vi "GetCalibData.vi"(8 "error in (no error)":errorcluster, 11 "BME68x in":refnum<class "BME680.lvclass">) -> (0 "error out":errorcluster, 3 "BME68x out":refnum<class "BME680.lvclass">)   [LabVIEW 2022 SP3, in "BME680.lvlib" / "BME680.lvclass"]
uses:
  BME680.lvclass
  BME680.lvclass/BME680.ctl
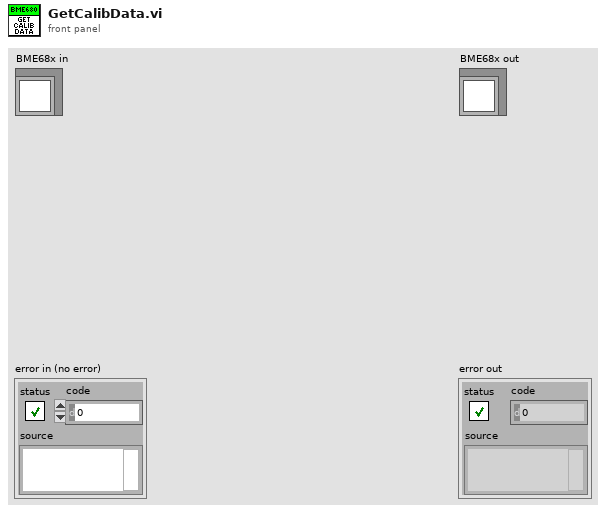
[diagram p1: front panel]
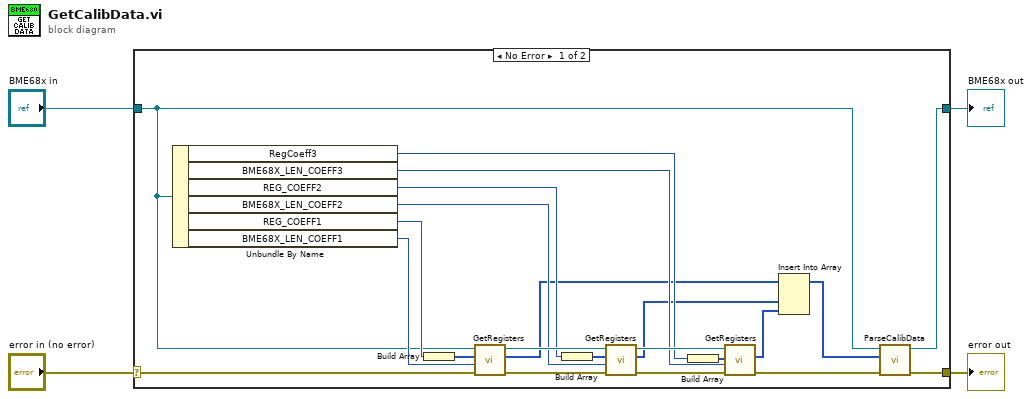
[diagram p0: block diagram]
diagram:
  n1 = case shown="No Error" "error in (no error)" {
    selector: "error in (no error)" -> [w26 w28]
    tunnel: [w11 w28] -> w3
    tunnel: [w5 w27] -> w1
    tunnel: "BME68x in" -> [w6 w27]
    frame No Error {
      n2 = Unbundle By Name(w6) -> ("RegCoeff3"=w15:u8, "BME68X_LEN_COEFF3"=w13:u8, "REG_COEFF2"=w18:u8, "BME68X_LEN_COEFF2"=w17:u8, "REG_COEFF1"=w24:u8, "BME68X_LEN_COEFF1"=w25:u8)
      n3 = Build Array(w24) -> (w23:u8[])
      n4 = call-dynamic "GetRegisters.vi"("error in (no error)"=w26, "Lenght"=w25, "Addr"=w23, "BME680 in"=w6) -> ("error out"=w22:errorcluster, "Data out"=w10:u8[], "BME680 out"=w20:refnum<class "BME680.lvclass">)  [unwired: 5 in]
      n5 = Build Array(w18) -> (w16:u8[])
      n6 = call-dynamic "GetRegisters.vi"("error in (no error)"=w22, "Lenght"=w17, "Addr"=w16, "BME680 in"=w20) -> ("error out"=w21:errorcluster, "Data out"=w8:u8[], "BME680 out"=w19:refnum<class "BME680.lvclass">)  [unwired: 5 in]
      n7 = Build Array(w15) -> (w14:u8[])
      n8 = call-dynamic "GetRegisters.vi"("error in (no error)"=w21, "Lenght"=w13, "Addr"=w14, "BME680 in"=w19) -> ("error out"=w12:errorcluster, "Data out"=w9:u8[])  [unwired: 5 in, 1 out]
      n9 = Insert Into Array(array=w10, new element #1=w8, new element #2=w9) -> (w7:u8[])  [unwired: 1 in]
      n10 = call "ParseCalibData.vi"("error in (no error)"=w12, "Calib Registers"=w7, "BME680 in"=w6) -> ("error out"=w11:errorcluster, "BME680 out"=w5:refnum<class "BME680.lvclass">)  [unwired: 7 in]
    }
    frame Error {
    }
  }
  "error out" <- w3
  "BME68x out" <- w1
